vi "P-541 Send Command.vi"(0 "VISA Ref":refnum<visa-resource-name>, 2 "Wait for Reply?":bool, 7 "Error In":errorcluster, 11 "Command":string) -> (4 "VISA Ref Out":refnum<visa-resource-name>, 8 "Error Out":errorcluster, 15 "Response":string)   [LabVIEW 2016]
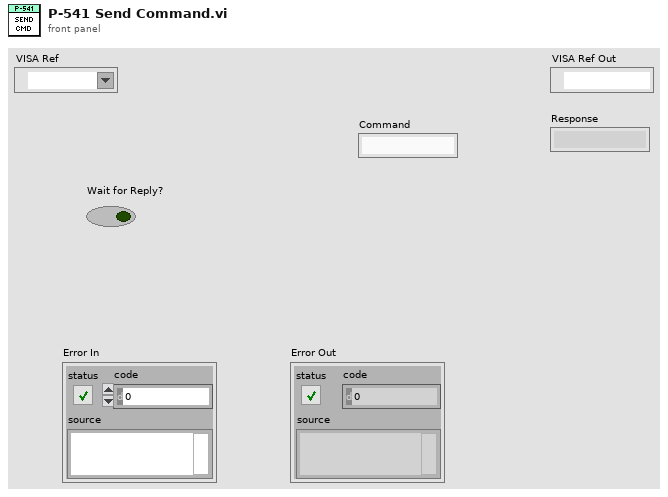
[diagram p1: front panel]
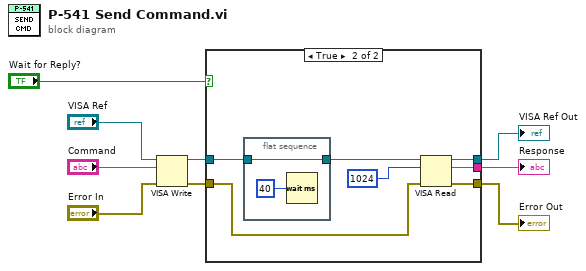
[diagram p0: block diagram]
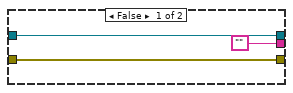
[diagram p2: hidden frame]
diagram:
  n1 = VISA Write(VISA resource name="VISA Ref", write buffer="Command", error in (no error)="Error In") -> (VISA resource name out=w9:refnum<visa-resource-name>, error out=w8:errorcluster)  [unwired: 1 out]
  n2 = case shown="True" "Wait for Reply?" {
    tunnel: w9 -> [w12 w19]
    tunnel: w8 -> [w11 w15]
    tunnel: [w12 w18] -> w6
    tunnel: [w11 w17] -> w5
    tunnel: ["" w16] -> w3
    frame False {
    }
    frame True {
      n3 = flat-sequence {
        tunnel: [w20] -> w14
        tunnel: w19 -> [w20]
        frame #0 {
          n4 = Wait (ms)(milliseconds to wait=u32 40) -> ()  [unwired: 1 out]
        }
      }
      n5 = VISA Read(VISA resource name=w14, byte count=u32 1024, error in (no error)=w15) -> (VISA resource name out=w18:refnum<visa-resource-name>, read buffer=w16:string, error out=w17:errorcluster)  [unwired: 1 out]
    }
  }
  "Response" <- w3
  "VISA Ref Out" <- w6
  "Error Out" <- w5
